vi "Config Reference Format.vi"(8 "error in":errorcluster, 9 "Loss Percent (off)":bool, 10 "Capacitance Percent (off)":bool, 11 "VISA resource name":refnum<visa-resource-name>) -> (0 "error out":errorcluster, 3 "VISA resource name out":refnum<visa-resource-name>)   [LabVIEW 2016, in "Andeen-Hagerling 2550.lvlib"]
doc: "This VI selects whether Reference result mode reports simple differences or percent differences."
uses:
  Andeen-Hagerling 2550.lvlib
panel:
  # "Reference Format"
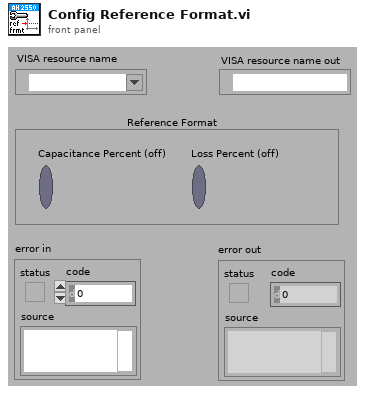
[diagram p1: front panel]
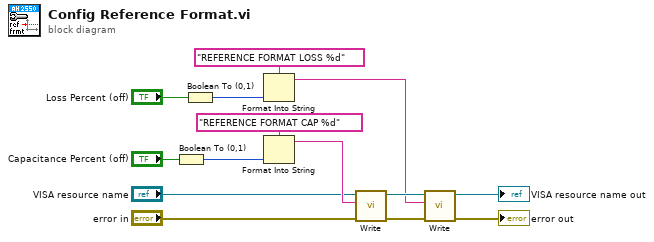
[diagram p0: block diagram]
diagram:
  n1 = Boolean To (0,1)(Boolean="Capacitance Percent (off)") -> (0, 1=w9:i16)
  n2 = Boolean To (0,1)(Boolean="Loss Percent (off)") -> (0, 1=w7:i16)
  n3 = Format Into String(format string="REFERENCE FORMAT LOSS %d", w7) -> (resulting string=w1:string)  [unwired: 2 in, 1 out]
  n4 = Format Into String(format string="REFERENCE FORMAT CAP %d", w9) -> (resulting string=w14:string)  [unwired: 2 in, 1 out]
  n5 = call "Write.vi"("error in"="error in", "command"=w14, "VISA resource name"="VISA resource name") -> ("error out"=w3:errorcluster, "VISA resource name out"=w5:refnum<visa-resource-name>)  [unwired: 7 in]
  n6 = call "Write.vi"("error in"=w3, "command"=w1, "VISA resource name"=w5) -> ("error out"=→"error out":errorcluster, "VISA resource name out"=→"VISA resource name out":refnum<visa-resource-name>)  [unwired: 7 in]
